vi "start Image Execution.vi"(8 "error in":errorcluster, 10 "imageId":u32, 11 "cycloneHandle":u32) -> (0 "error out":errorcluster, 3 "function return":bool)   [LabVIEW 2021, in "CycloneControlSDK.lvlib"]
doc: "extern \"C\" bool _cdecl startImageExecution(uint32_t cycloneHandle, uint32_t imageId);"
uses:
  CycloneControlSDK.lvlib
  CycloneControlSDK_64.dll
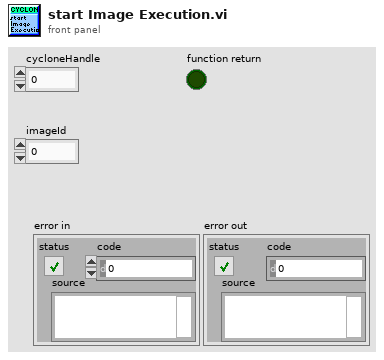
[diagram p1: front panel]
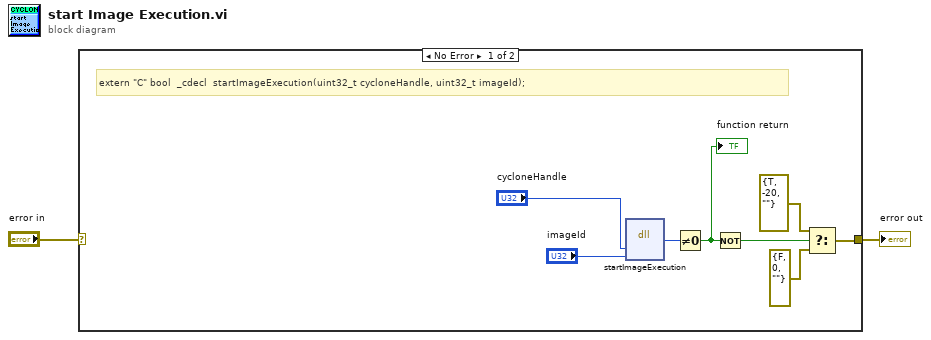
[diagram p0: block diagram]
diagram:
  n1 = case shown="No Error" "error in" {
    selector: "error in" -> [_ w11]
    tunnel: [w5 w11] -> w1
    frame No Error {
      # "extern \"C\" bool\t\t_cdecl  startImageExecution(uint32_t cycloneHandle, uint32_t imageId);"
      n2 = dll-call lib="C:/PEMicro/cyclone/cycloneControl/controlsdk/examples/labview2018/user.lib/CycloneControlSDK/CycloneControlSDK_64.dll" fn="startImageExecution"("cycloneHandle"="cycloneHandle", "imageId"="imageId") -> ("return type"=w10:u8)  [unwired: 5 in, 2 out]
      n3 = Not Equal To 0?(x=w10) -> (x != 0?=w4:bool)
      "function return" <- w4
      n4 = Not(x=w4) -> (.not. x?=w3:bool)
      n5 = Select(t=errorcluster {"status"=TRUE, "code"=-20, "source"=""} ("error constant"), s=w3, f=errorcluster {"status"=FALSE, "code"=0, "source"=""} ("error constant")) -> (s? t:f=w5:errorcluster)
    }
    frame Error {
    }
  }
  "error out" <- w1
